vi "Set Invoke __Output.vi"(7 "Complete Call (T)":bool=TRUE, 8 "error in (no error)":errorcluster, 10 "Message_Data":T1, 11 "gRPCid":T2) -> (0 "error out":errorcluster)   [LabVIEW 2019, in "OOP Server.lvlib" / "OOP Server.lvclass"]
uses:
  gRPC interface/Server API/typeDefs/grpcId.ctl
  <vilib>/Utility/error.llb/Error Cluster From Error Code.vi
  OOP Server.lvclass
  gRPC interface/gprc-lvsupport.lvlib
  RPC Messages/InvokeResponse/InvokeResponse_Data.ctl
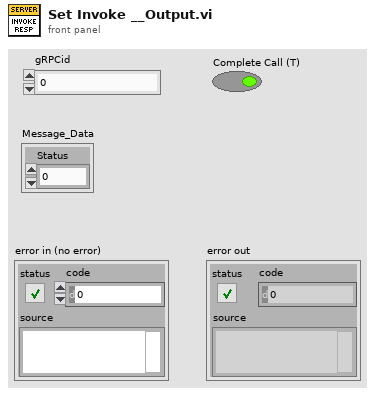
[diagram p1: front panel]
types:
  T1 = typedef "OOP Server.lvlib/OOP Server.lvclass/InvokeResponse_Data.ctl" = cluster{"Status":i32}
  T2 = typedef "gprc-lvsupport.lvlib/grpcId.ctl" = u64
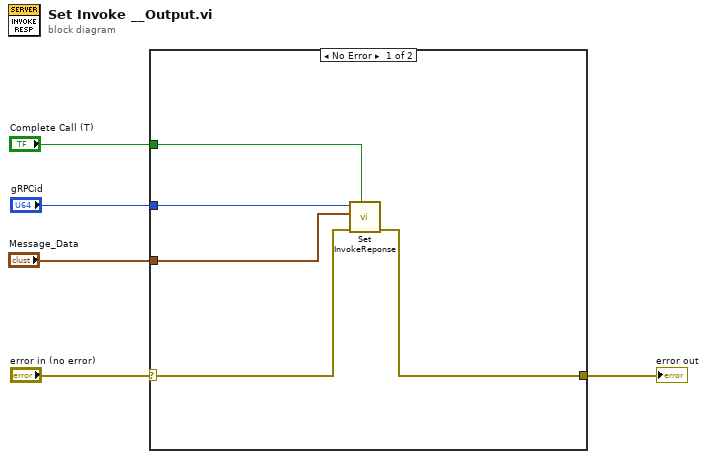
[diagram p0: block diagram]
diagram:
  n1 = case shown="No Error" "error in (no error)" {
    selector: "error in (no error)" -> [w9 w11]
    tunnel: "gRPCid" -> [w10 _]
    tunnel: [w8 w11] -> w3
    tunnel: "Complete Call (T)" -> [w7 _]
    tunnel: "Message_Data" -> [w6 _]
    frame No Error {
      n2 = call "Set InvokeReponse.vi"("Complete Call (T)"=w7, "error in (no error)"=w9, "InvokeResponse_Data"=w6, "gRPCid"=w10) -> ("error out"=w8:errorcluster)  [unwired: 7 in]
    }
    frame Error {
    }
  }
  "error out" <- w3
